vi "UDP - Write Data.vi"(7 "V2":bool, 10 "Data":T2={"Test"={"Target Load"=0.0, "Target Disp"=0.0, "Rate"=0.0, "Speed"=0.0}, "Sensor"={"Name"=[], "Unit"=[], "Decimal Point"=[], "Ch Log"=[], "H Alarm"=[], "L Alarm"=[], "H Limit"=[], "L Limit"=[], "Filter"=[], "Gain"=[], "Calib Type"=[]}, "PID"={"SP"=0.0, "PV"=0.0, "kP"=0.0, "kI"=0.0, "kD"=0.0, "FF"=0.0, "Err Band"=0.0, "Max"=0, "Min"=0, "Ts"=0, "Out"=0, "Mode"=0}, "ADC"={"Active Ch"=[], "Filter Type"=0, "Post Filter"=[], "Gain"=[], "FS"=0, "IntOC"=0, "IntFC"=0, "SysOC"=0, "Cofficient"=[], "K"=[], "Max"=0}, "System"={"Out Type"=0, "Inverse"=0, "Monitor"=0, "Reserve"=0, "ACC Time"=0, "Pulse Rev"=0, "Stroke"=0, "Auto Off"=0, "Gear Ratio"=0.0, "Pitch"=0.0, "Max Speed"=0, "Jog Speed"=0, "Disp Coff"=0.0, "Max Load"=0}, "Index"=enum."Ch1", "Datalog"=enum."Empty"}, 11 "CMD":T1) -> (3 "Array":u8[](array[numeric]))   [LabVIEW 2019]
uses:
  Controls/Communication - Write Data.ctl
  Controls/UDP - Command.ctl
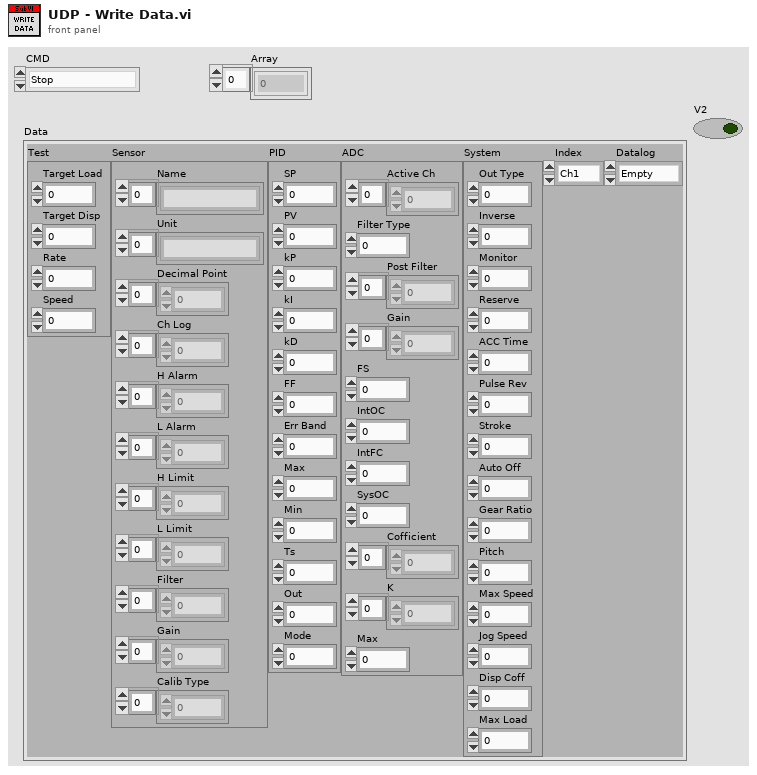
[diagram p1: front panel]
types:
  T1 = typedef "UDP - Command.ctl" = enum16{"Stop", "Jog Up", "Jog Down", "Ramp Up", "Ramp Down", "PID Target", "PID Ramp", "Disp Run", "Read Ch Data", "Zero Channel", "Zero Disp", "Read Sensor", "Write Sensor", "Read ADC", "Write ADC", "Read PID", "Write PID", "Read Test", "Write Test", "Read System", "Write System", "Read Datalog", "Read Datalog Sensor"}
  T2 = typedef "Communication - Write Data.ctl" = cluster{"Test":cluster{"Target Load":sgl, "Target Disp":sgl, "Rate":sgl, "Speed":sgl}, "Sensor":cluster{"Name":string[], "Unit":string[], "Decimal Point":u8[], "Ch Log":u8[], "H Alarm":u8[], "L Alarm":u8[], "H Limit":sgl[], "L Limit":sgl[], "Filter":u8[], "Gain":u8[], "Calib Type":u32[]}, "PID":cluster{"SP":sgl, "PV":sgl, "kP":sgl, "kI":sgl, "kD":sgl, "FF":sgl, "Err Band":sgl, "Max":i32, "Min":i32, "Ts":u32, "Out":i32, "Mode":u8}, "ADC":cluster{"Active Ch":u8[], "Filter Type":u8, "Post Filter":u8[], "Gain":u8[], "FS":u16, "IntOC":u8, "IntFC":u8, "SysOC":u8, "Cofficient":dbl[], "K":dbl[], "Max":i32}, "System":cluster{"Out Type":u8, "Inverse":u8, "Monitor":u8, "Reserve":u8, "ACC Time":u32, "Pulse Rev":u32, "Stroke":u32, "Auto Off":u32, "Gear Ratio":sgl, "Pitch":sgl, "Max Speed":u32, "Jog Speed":u32, "Disp Coff":sgl, "Max Load":u32}, "Index":enum16{"Ch1", "Ch2", "Ch3", "Ch4", "Ch5", "Ch6", "Ch7", "Ch8", "Ch9", "Ch10", "Ch11", "Ch12", "Ch13", "Ch14", "Ch15", "Ch16"}, "Datalog":enum16{"Ch1-Ch16", "Ch17-Ch32", "Ch32-Ch48", "Ch49-Ch64", "Empty"}}
  T3 = enum16{"Ch1-Ch16", "Ch17-Ch32", "Ch32-Ch48", "Ch49-Ch64", "Empty"}
  T4 = enum16{"Ch1", "Ch2", "Ch3", "Ch4", "Ch5", "Ch6", "Ch7", "Ch8", "Ch9", "Ch10", "Ch11", "Ch12", "Ch13", "Ch14", "Ch15", "Ch16"}
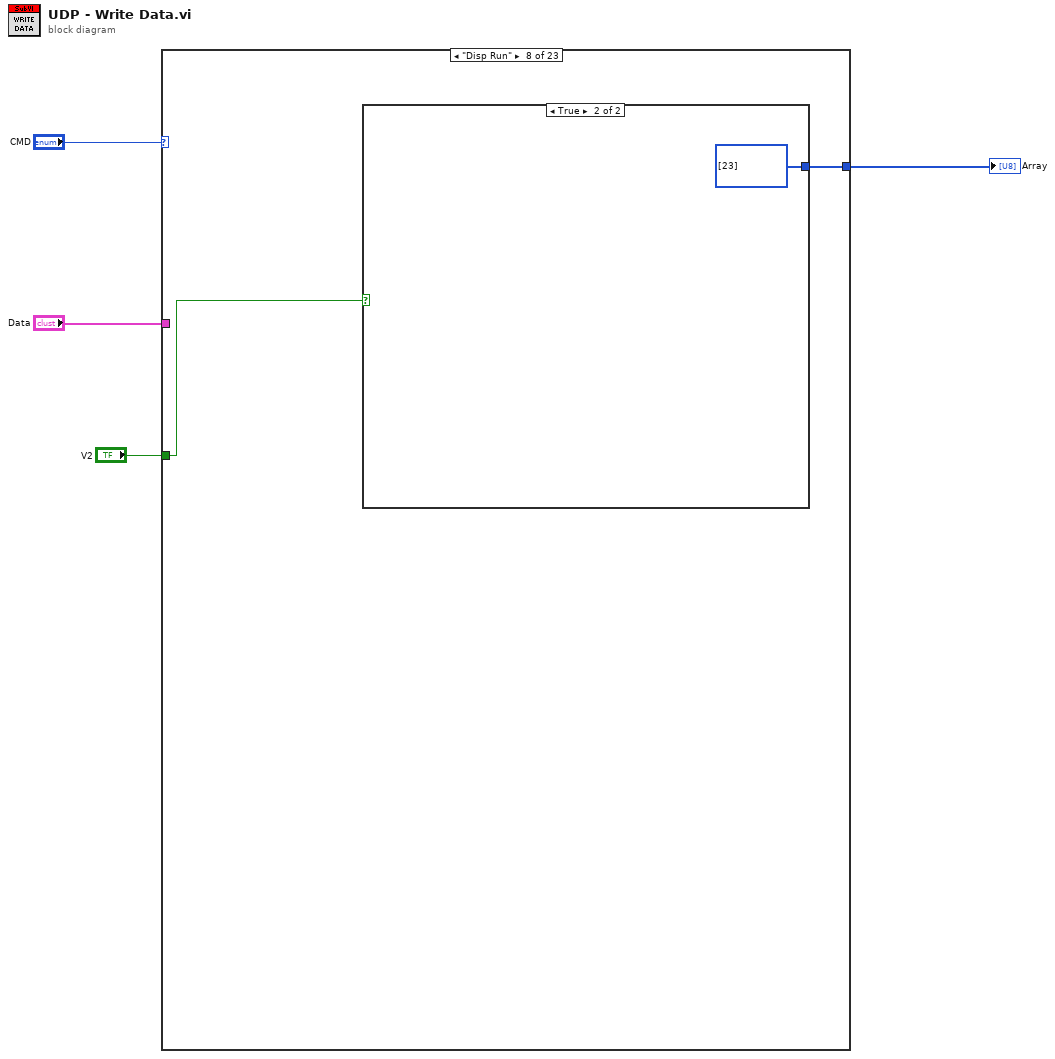
[diagram p0: block diagram]
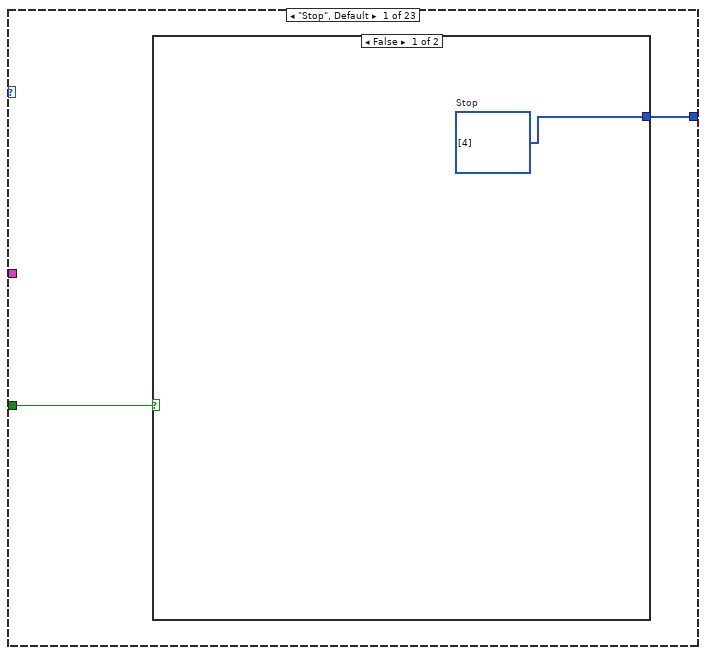
[diagram p2: hidden frame]
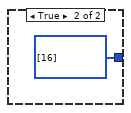
[diagram p3: hidden frame]
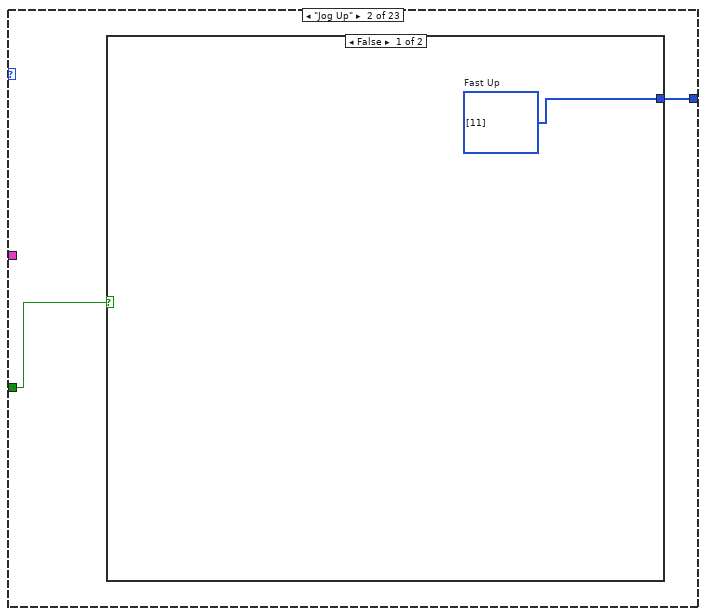
[diagram p4: hidden frame]
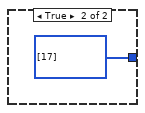
[diagram p5: hidden frame]
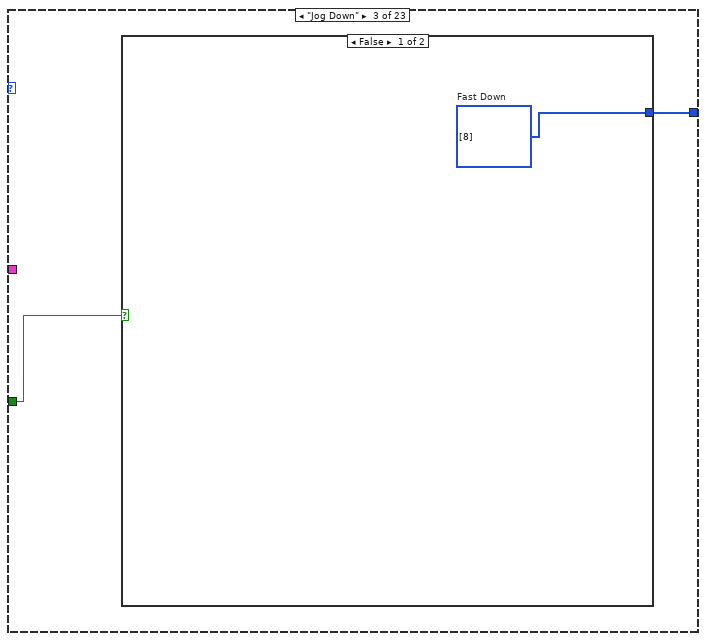
[diagram p6: hidden frame]
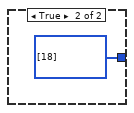
[diagram p7: hidden frame]
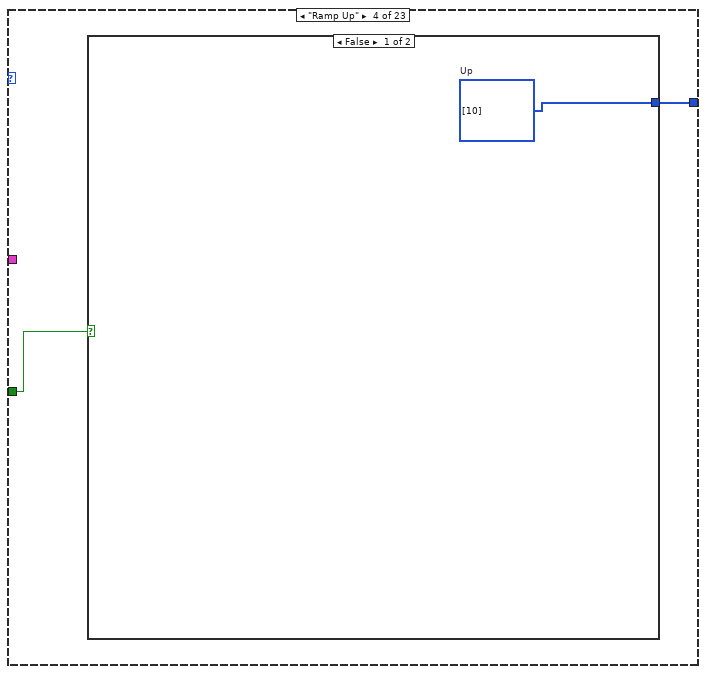
[diagram p8: hidden frame]
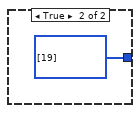
[diagram p9: hidden frame]
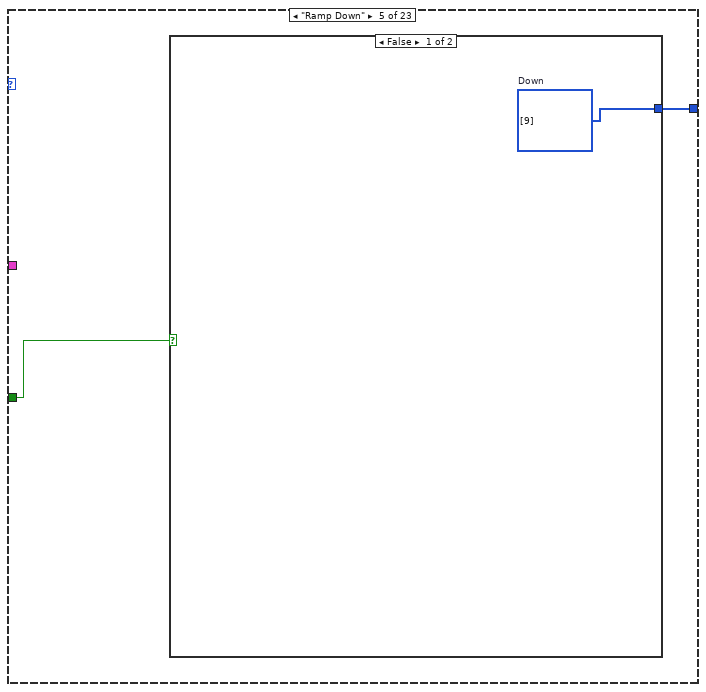
[diagram p10: hidden frame]
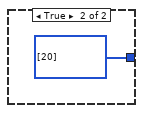
[diagram p11: hidden frame]
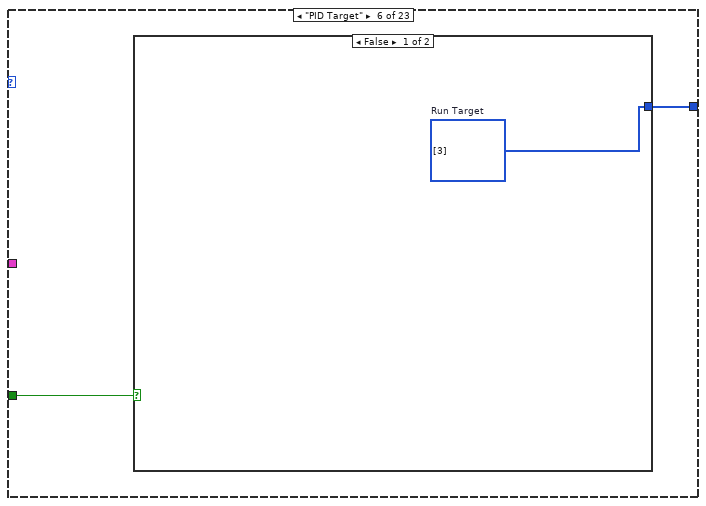
[diagram p12: hidden frame]
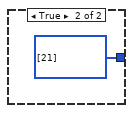
[diagram p13: hidden frame]
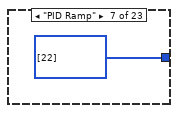
[diagram p14: hidden frame]
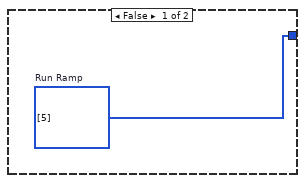
[diagram p15: hidden frame]
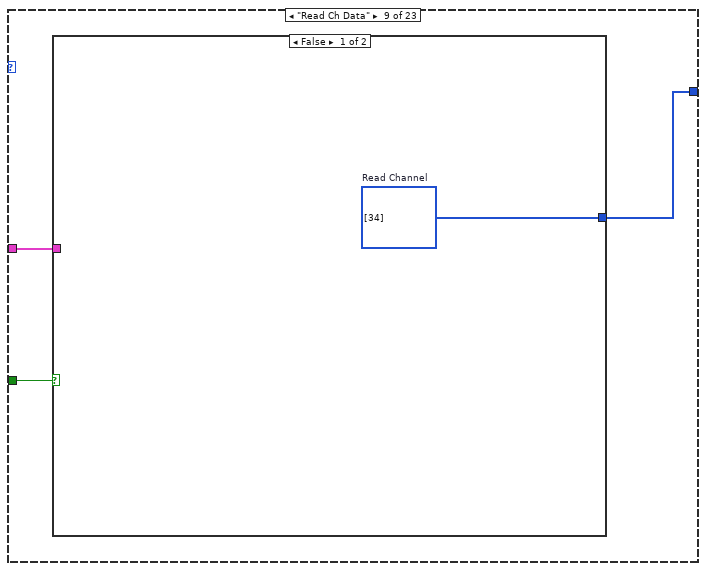
[diagram p16: hidden frame]
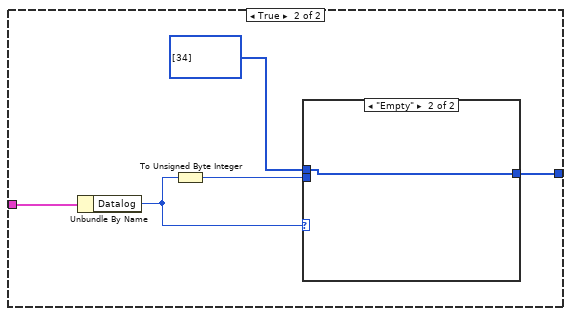
[diagram p17: hidden frame]
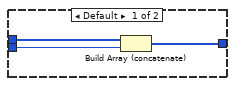
[diagram p18: hidden frame]
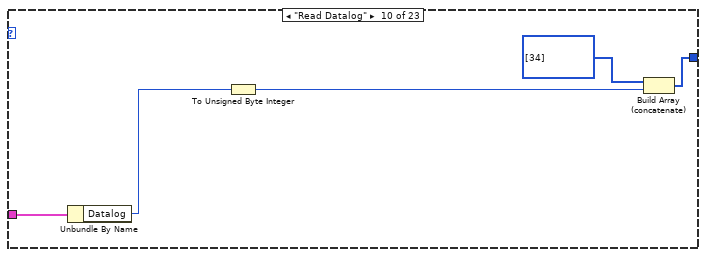
[diagram p19: hidden frame]
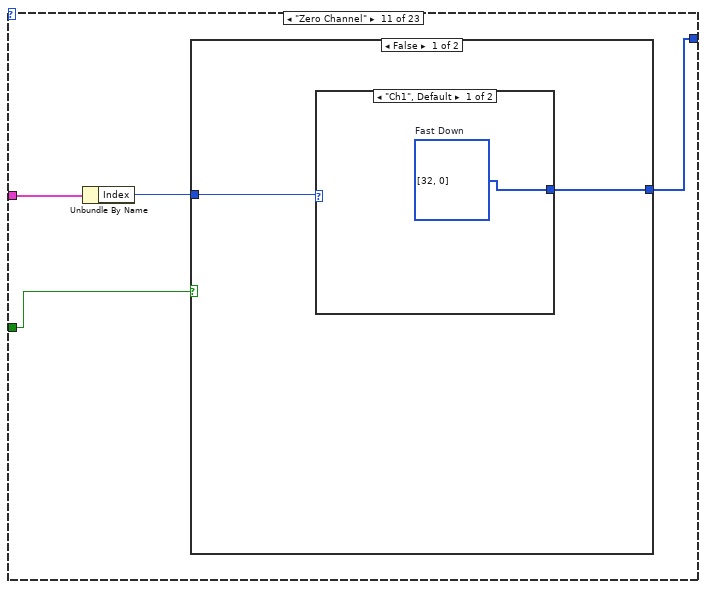
[diagram p20: hidden frame]
diagram:
  n1 = case shown="\"Disp Run\"" "CMD" {
    tunnel: [w6 w10 w14 w18 w22 w26 u8[] [22] w31 w35 w48 w55 w79 w83 w87 w91 u8[] [56] w155 u8[] [58] w237 u8[] [48] w241 u8[] [52] w282] -> w2
    tunnel: "Data" -> [_ _ _ _ _ _ _ _ w36 w51 w54 _ _ w89 w90 _ w154 _ w236 _ w240 _ w281]
    tunnel: "V2" -> [w5 w9 w13 w17 w21 w25 _ w30 w34 _ w52 w78 w82 _ _ _ _ _ _ _ w239 _ _]
    frame "Stop", Default {
      n2 = case shown="False" w5 {
        tunnel: [w7 u8[] [16]] -> w6
        frame False {
          w7 = u8[] [4]  # Stop
        }
        frame True {
        }
      }
    }
    frame "Jog Up" {
      n3 = case shown="False" w9 {
        tunnel: [w11 u8[] [17]] -> w10
        frame False {
          w11 = u8[] [11]  # Fast Up
        }
        frame True {
        }
      }
    }
    frame "Jog Down" {
      n4 = case shown="False" w13 {
        tunnel: [w15 u8[] [18]] -> w14
        frame False {
          w15 = u8[] [8]  # Fast Down
        }
        frame True {
        }
      }
    }
    frame "Ramp Up" {
      n5 = case shown="False" w17 {
        tunnel: [w19 u8[] [19]] -> w18
        frame False {
          w19 = u8[] [10]  # Up
        }
        frame True {
        }
      }
    }
    frame "Ramp Down" {
      n6 = case shown="False" w21 {
        tunnel: [w23 u8[] [20]] -> w22
        frame False {
          w23 = u8[] [9]  # Down
        }
        frame True {
        }
      }
    }
    frame "PID Target" {
      n7 = case shown="False" w25 {
        tunnel: [w27 u8[] [21]] -> w26
        frame False {
          w27 = u8[] [3]  # Run Target
        }
        frame True {
        }
      }
    }
    frame "PID Ramp" {
    }
    frame "Disp Run" {
      n8 = case shown="True" w30 {
        tunnel: [w32 u8[] [23]] -> w31
        frame False {
          w32 = u8[] [5]  # Run Ramp
        }
        frame True {
        }
      }
    }
    frame "Read Ch Data" {
      n9 = case shown="False" w34 {
        tunnel: w36 -> [_ w42]
        tunnel: [w37 w40] -> w35
        frame False {
          w37 = u8[] [34]  # Read Channel
        }
        frame True {
          n10 = Unbundle By Name(w42) -> ("Datalog"=w38:T3)
          n11 = To Unsigned Byte Integer(number=w38) -> (unsigned 8bit integer=w39:u8)
          n12 = case shown="\"Empty\"" w38 {
            tunnel: w39 -> [w45 _]
            tunnel: u8[] [34] -> [w44 w46]
            tunnel: [w43 w46] -> w40
            frame Default {
              n13 = Build Array (concatenate)(w44, w45) -> (w43:u8[])
            }
            frame "Empty" {
            }
          }
        }
      }
    }
    frame "Read Datalog" {
      n14 = Unbundle By Name(w51) -> ("Datalog"=w50:T3)
      n15 = To Unsigned Byte Integer(number=w50) -> (unsigned 8bit integer=w47:u8)
      n16 = Build Array (concatenate)(u8[] [34], w47) -> (w48:u8[])
    }
    frame "Zero Channel" {
      n17 = Unbundle By Name(w54) -> ("Index"=w53:T4)
      n18 = case shown="False" w52 {
        tunnel: [w57 w61] -> w55
        tunnel: w53 -> [w56 w60]
        frame False {
          n19 = case shown="\"Ch1\", Default" w56 {
            tunnel: [w58 w59] -> w57
            frame "Ch1", Default {
              w58 = u8[] [32, 0]  # Fast Down
            }
            frame "Ch2" {
              w59 = u8[] [32, 1]  # Fast Down
            }
          }
        }
        frame True {
          n20 = case shown="\"Ch6\"" w60 {
            tunnel: [u8[] [32, 0] u8[] [32, 1] u8[] [32, 2] u8[] [32, 3] u8[] [32, 4] u8[] [32, 5] u8[] [32, 6] u8[] [32, 7] u8[] [32, 8] u8[] [32, 9] u8[] [32, 10] u8[] [32, 11] u8[] [32, 12] u8[] [32, 13] u8[] [32, 14] u8[] [32, 15]] -> w61
            frame "Ch1", Default {
            }
            frame "Ch2" {
            }
            frame "Ch3" {
            }
            frame "Ch4" {
            }
            frame "Ch5" {
            }
            frame "Ch6" {
            }
            frame "Ch7" {
            }
            frame "Ch8" {
            }
            frame "Ch9" {
            }
            frame "Ch10" {
            }
            frame "Ch11" {
            }
            frame "Ch12" {
            }
            frame "Ch13" {
            }
            frame "Ch14" {
            }
            frame "Ch15" {
            }
            frame "Ch16" {
            }
          }
        }
      }
    }
    frame "Zero Disp" {
      n21 = case shown="False" w78 {
        tunnel: [w80 u8[] [33]] -> w79
        frame False {
          w80 = u8[] [33]  # Fast Down
        }
        frame True {
        }
      }
    }
    frame "Read Sensor" {
      n22 = case shown="False" w82 {
        tunnel: [w84 u8[] [60]] -> w83
        frame False {
          w84 = u8[] [52]  # Read Unit
        }
        frame True {
        }
      }
    }
    frame "Read Datalog Sensor" {
      n23 = Unbundle By Name(w89) -> ("Index"=w86:T4)
      n24 = Build Array (concatenate)(u8[] [50], w86) -> (w87:u16[])
    }
    frame "Write Sensor" {
      n25 = Unbundle By Name(w90) -> ("Sensor.Name"=w96:string[], "Sensor.Unit"=w95:string[], "Sensor.Decimal Point"=w94:u8[], "Sensor.Ch Log"=w93:u8[], "Sensor.H Alarm"=w97:u8[], "Sensor.L Alarm"=w98:u8[], "Sensor.H Limit"=w99:sgl[], "Sensor.L Limit"=w100:sgl[], "Sensor.Filter"=w101:u8[], "Sensor.Gain"=w102:u8[], "Sensor.Calib Type"=w103:u32[])
      n26 = for {
        tunnel: w93 -> [w144] mode=indexing
        tunnel: w94 -> [w143] mode=indexing
        tunnel: w95 -> [w111] mode=indexing
        tunnel: w96 -> [w122] mode=indexing
        tunnel: w97 -> [w132] mode=indexing
        tunnel: w98 -> [w131] mode=indexing
        tunnel: w99 -> [w130] mode=indexing
        tunnel: w100 -> [w129] mode=indexing
        tunnel: w101 -> [w128] mode=indexing
        tunnel: w102 -> [w127] mode=indexing
        tunnel: w103 -> [w126] mode=indexing
        tunnel: [w123] -> w104 mode=concatenating
        w133 = u8[] []
        n27 = String Length(string=w122) -> (length=w120:i32)
        n28 = String Length(string=w111) -> (length=w113:i32)
        n29 = Subtract(x=10, y=w120) -> (x-y=w119:i32)
        n30 = Subtract(x=6, y=w113) -> (x-y=w114:i32)
        n31 = Type Cast(type=w133, x=w122) -> (*(type *) &x=w116:u8[])
        n32 = Type Cast(type=w133, x=w111) -> (*(type *) &x=w110:u8[])
        n33 = Type Cast(type=w133, x=w143) -> (*(type *) &x=w142:u8[])
        n34 = Type Cast(type=w133, x=w144) -> (*(type *) &x=w141:u8[])
        n35 = Type Cast(type=w133, x=w132) -> (*(type *) &x=w137:u8[])
        n36 = Type Cast(type=w133, x=w131) -> (*(type *) &x=w138:u8[])
        n37 = Type Cast(type=w133, x=w130) -> (*(type *) &x=w139:u8[])
        n38 = Type Cast(type=w133, x=w129) -> (*(type *) &x=w140:u8[])
        n39 = Type Cast(type=w133, x=w128) -> (*(type *) &x=w136:u8[])
        n40 = Type Cast(type=w133, x=w127) -> (*(type *) &x=w135:u8[])
        n41 = Type Cast(type=w133, x=w126) -> (*(type *) &x=w134:u8[])
        n42 = Initialize Array(u8 0 ("Numeric"), w119) -> (w117:u8[])
        n43 = Initialize Array(u8 0 ("Numeric"), w114) -> (w108:u8[])
        n44 = Reverse 1D Array(array=w139) -> (reversed array=w125:u8[])
        n45 = Reverse 1D Array(array=w140) -> (reversed array=w124:u8[])
        n46 = Reverse 1D Array(array=w134) -> (reversed array=w106:u8[])
        n47 = Build Array (concatenate)(w116, w117) -> (w109:u8[])
        n48 = Build Array (concatenate)(w110, w108) -> (w107:u8[])
        n49 = Build Array (concatenate)(w109, w107, w142, w141, w137, w138, w125, w124, w136, w135, u8[] [0, 0] ("array"), w106) -> (w123:u8[])
      }
      n50 = Build Array (concatenate)(u8[] [61], w104) -> (w91:u8[])
    }
    frame "Read ADC" {
    }
    frame "Write ADC" {
      w158 = u8[] []
      n51 = Unbundle By Name(w154) -> ("ADC.Active Ch"=w160:u8[], "ADC.Filter Type"=w161:u8, "ADC.Post Filter"=w162:u8[], "ADC.Gain"=w163:u8[], "ADC.FS"=w164:u16, "ADC.IntOC"=w165:u8, "ADC.IntFC"=w166:u8, "ADC.SysOC"=w167:u8, "ADC.Cofficient"=w168:dbl[], "ADC.K"=w147:dbl[], "ADC.Max"=w169:i32)
      n52 = Number To Fractional String(number=w147, precision (6)=i16 4) -> (F-format string=w148:string[])  [unwired: 2 in]
      n53 = Fract/Exp String To Number(string=w148) -> (number=w146:dbl[])  [unwired: 3 in, 1 out]
      n54 = for {
        tunnel: [w195] -> w170 mode=concatenating
        tunnel: w160 -> [w194] mode=indexing
        n55 = Type Cast(type=u8[] [], x=w194) -> (*(type *) &x=w195:u8[])
      }
      n56 = for {
        tunnel: [w192] -> w172 mode=concatenating
        tunnel: w162 -> [w191] mode=indexing
        n57 = Type Cast(type=u8[] [], x=w191) -> (*(type *) &x=w192:u8[])
      }
      n58 = for {
        tunnel: [w189] -> w173 mode=concatenating
        tunnel: w163 -> [w188] mode=indexing
        n59 = Type Cast(type=u8[] [], x=w188) -> (*(type *) &x=w189:u8[])
      }
      n60 = for {
        tunnel: [w184] -> w152 mode=concatenating
        tunnel: w168 -> [w186] mode=indexing
        n61 = Type Cast(type=u8[] [], x=w186) -> (*(type *) &x=w185:u8[])
        n62 = Reverse 1D Array(array=w185) -> (reversed array=w184:u8[])
      }
      n63 = for {
        tunnel: [w180] -> w178 mode=concatenating
        tunnel: w146 -> [w182] mode=indexing
        n64 = Type Cast(type=u8[] [], x=w182) -> (*(type *) &x=w181:u8[])
        n65 = Reverse 1D Array(array=w181) -> (reversed array=w180:u8[])
      }
      n66 = Type Cast(type=u8[] [], x=w161) -> (*(type *) &x=w171:u8[])
      n67 = Type Cast(type=w158, x=w164) -> (*(type *) &x=w174:u8[])
      n68 = Type Cast(type=w158, x=w165) -> (*(type *) &x=w175:u8[])
      n69 = Type Cast(type=w158, x=w166) -> (*(type *) &x=w176:u8[])
      n70 = Type Cast(type=w158, x=w167) -> (*(type *) &x=w177:u8[])
      n71 = Type Cast(type=u8[] [], x=w169) -> (*(type *) &x=w153:u8[])
      n72 = Reverse 1D Array(array=w153) -> (reversed array=w150:u8[])
      n73 = Build Array (concatenate)(w170, w171, w172, w173, w174, w175, w176, w177, u8[] [63, 0] ("array"), w152, w178, w150) -> (w179:u8[])
      n74 = Build Array (concatenate)(u8[] [57], w179) -> (w155:u8[])
    }
    frame "Read PID" {
    }
    frame "Write PID" {
      w218 = u8[] []
      n75 = Unbundle By Name(w236) -> ("PID.SP"=w201:sgl, "PID.PV"=w200:sgl, "PID.kP"=w199:sgl, "PID.kI"=w198:sgl, "PID.kD"=w219:sgl, "PID.FF"=w220:sgl, "PID.Err Band"=w221:sgl, "PID.Max"=w222:i32, "PID.Min"=w223:i32, "PID.Ts"=w224:u32, "PID.Out"=w225:i32, "PID.Mode"=w226:u8)
      n76 = Type Cast(type=w218, x=w201) -> (*(type *) &x=w202:u8[])
      n77 = Type Cast(type=w218, x=w200) -> (*(type *) &x=w203:u8[])
      n78 = Type Cast(type=w218, x=w199) -> (*(type *) &x=w204:u8[])
      n79 = Type Cast(type=w218, x=w198) -> (*(type *) &x=w205:u8[])
      n80 = Type Cast(type=w218, x=w219) -> (*(type *) &x=w214:u8[])
      n81 = Type Cast(type=w218, x=w220) -> (*(type *) &x=w213:u8[])
      n82 = Type Cast(type=w218, x=w221) -> (*(type *) &x=w212:u8[])
      n83 = Type Cast(type=w218, x=w222) -> (*(type *) &x=w211:u8[])
      n84 = Type Cast(type=w218, x=w223) -> (*(type *) &x=w215:u8[])
      n85 = Type Cast(type=w218, x=w224) -> (*(type *) &x=w216:u8[])
      n86 = Type Cast(type=w218, x=w225) -> (*(type *) &x=w217:u8[])
      n87 = Type Cast(type=w218, x=w226) -> (*(type *) &x=w234:u8[])
      n88 = Reverse 1D Array(array=w202) -> (reversed array=w206:u8[])
      n89 = Reverse 1D Array(array=w203) -> (reversed array=w207:u8[])
      n90 = Reverse 1D Array(array=w204) -> (reversed array=w208:u8[])
      n91 = Reverse 1D Array(array=w205) -> (reversed array=w209:u8[])
      n92 = Reverse 1D Array(array=w214) -> (reversed array=w227:u8[])
      n93 = Reverse 1D Array(array=w213) -> (reversed array=w228:u8[])
      n94 = Reverse 1D Array(array=w212) -> (reversed array=w229:u8[])
      n95 = Reverse 1D Array(array=w211) -> (reversed array=w230:u8[])
      n96 = Reverse 1D Array(array=w215) -> (reversed array=w231:u8[])
      n97 = Reverse 1D Array(array=w216) -> (reversed array=w232:u8[])
      n98 = Reverse 1D Array(array=w217) -> (reversed array=w233:u8[])
      n99 = Build Array (concatenate)(w206, w207, w208, w209, w227, w228, w229, w230, w231, w232, w233, w234) -> (w235:u8[])
      n100 = Build Array (concatenate)(u8[] [59], w235) -> (w237:u8[])
    }
    frame "Read Test" {
    }
    frame "Write Test" {
      n101 = case shown="False" w239 {
        tunnel: [w246 w270] -> w241
        tunnel: w240 -> [w245 w255]
        frame False {
          n102 = Unbundle By Name(w245) -> ("Test.Target Load"=w244:sgl, "Test.Speed"=w243:sgl)
          n103 = Equal To 0?(x=w243) -> (x = 0?=w242:bool)
          n104 = case shown="False" w242 {
            tunnel: [w248 w253] -> w246
            tunnel: w244 -> [w247 _]
            tunnel: w243 -> [_ w252]
            frame True {
              w250 = u8[] [6]  # Set Target
              n105 = call "FTDI - Float to Byte.vi"("Float"=w247) -> ("Byte"=w249:u8[])  [unwired: 10 in]
              n106 = Build Array (concatenate)(w250, w249) -> (w248:u8[])
            }
            frame False {
              w254 = u8[] [7]  # Set Ramp
              n107 = call "FTDI - Float to Byte.vi"("Float"=w252) -> ("Byte"=w251:u8[])  [unwired: 10 in]
              n108 = Build Array (concatenate)(w254, w251) -> (w253:u8[])
            }
          }
        }
        frame True {
          w261 = u8[] []
          n109 = Unbundle By Name(w255) -> ("Test.Target Load"=w259:sgl, "Test.Target Disp"=w258:sgl, "Test.Rate"=w257:sgl, "Test.Speed"=w256:sgl)
          n110 = Type Cast(type=w261, x=w259) -> (*(type *) &x=w262:u8[])
          n111 = Type Cast(type=w261, x=w258) -> (*(type *) &x=w263:u8[])
          n112 = Type Cast(type=w261, x=w257) -> (*(type *) &x=w264:u8[])
          n113 = Type Cast(type=w261, x=w256) -> (*(type *) &x=w265:u8[])
          n114 = Reverse 1D Array(array=w262) -> (reversed array=w266:u8[])
          n115 = Reverse 1D Array(array=w263) -> (reversed array=w267:u8[])
          n116 = Reverse 1D Array(array=w264) -> (reversed array=w268:u8[])
          n117 = Reverse 1D Array(array=w265) -> (reversed array=w269:u8[])
          n118 = Build Array (concatenate)(w266, w267, w268, w269) -> (w260:u8[])
          n119 = Build Array (concatenate)(u8[] [49], w260) -> (w270:u8[])
        }
      }
    }
    frame "Read System" {
    }
    frame "Write System" {
      w274 = u8[] []
      n120 = Unbundle By Name(w281) -> ("System.Out Type"=w286:u8, "System.Inverse"=w285:u8, "System.Monitor"=w284:u8, "System.Reserve"=w283:u8, "System.ACC Time"=w299:u32, "System.Pulse Rev"=w300:u32, "System.Stroke"=w301:u32, "System.Auto Off"=w302:u32, "System.Gear Ratio"=w303:sgl, "System.Pitch"=w304:sgl, "System.Max Speed"=w305:u32, "System.Jog Speed"=w306:u32, "System.Disp Coff"=w277:sgl, "System.Max Load"=w276:u32)
      n121 = Type Cast(type=w274, x=w286) -> (*(type *) &x=w287:u8[])
      n122 = Type Cast(type=w274, x=w285) -> (*(type *) &x=w288:u8[])
      n123 = Type Cast(type=w274, x=w284) -> (*(type *) &x=w289:u8[])
      n124 = Type Cast(type=w274, x=w283) -> (*(type *) &x=w290:u8[])
      n125 = Type Cast(type=w274, x=w299) -> (*(type *) &x=w295:u8[])
      n126 = Type Cast(type=w274, x=w300) -> (*(type *) &x=w294:u8[])
      n127 = Type Cast(type=w274, x=w301) -> (*(type *) &x=w293:u8[])
      n128 = Type Cast(type=w274, x=w302) -> (*(type *) &x=w292:u8[])
      n129 = Type Cast(type=w274, x=w303) -> (*(type *) &x=w296:u8[])
      n130 = Type Cast(type=w274, x=w304) -> (*(type *) &x=w297:u8[])
      n131 = Type Cast(type=w274, x=w305) -> (*(type *) &x=w298:u8[])
      n132 = Type Cast(type=w274, x=w306) -> (*(type *) &x=w314:u8[])
      n133 = Type Cast(type=w274, x=w277) -> (*(type *) &x=w279:u8[])
      n134 = Type Cast(type=w274, x=w276) -> (*(type *) &x=w278:u8[])
      n135 = Reverse 1D Array(array=w295) -> (reversed array=w307:u8[])
      n136 = Reverse 1D Array(array=w294) -> (reversed array=w308:u8[])
      n137 = Reverse 1D Array(array=w293) -> (reversed array=w309:u8[])
      n138 = Reverse 1D Array(array=w292) -> (reversed array=w310:u8[])
      n139 = Reverse 1D Array(array=w296) -> (reversed array=w311:u8[])
      n140 = Reverse 1D Array(array=w297) -> (reversed array=w312:u8[])
      n141 = Reverse 1D Array(array=w298) -> (reversed array=w313:u8[])
      n142 = Reverse 1D Array(array=w314) -> (reversed array=w280:u8[])
      n143 = Reverse 1D Array(array=w279) -> (reversed array=w275:u8[])
      n144 = Reverse 1D Array(array=w278) -> (reversed array=w273:u8[])
      n145 = Build Array (concatenate)(w287, w288, w289, w290, w307, w308, w309, w310, w311, w312, w313, w280, w275, w273) -> (w315:u8[])
      n146 = Build Array (concatenate)(u8[] [53], w315) -> (w282:u8[])
    }
  }
  "Array" <- w2
